vi "SavePixelsVals.vi"(0 "ROI Coordinates out":T1, 5 "Pixel SizeX":dbl, 6 "3D out":T2, 7 "Pixel SizeY":dbl, 8 "Stack length":dbl, 9 "X Start":dbl, 10 "Stack Start":dbl, 11 "error out 2":errorcluster, 12 "X length":dbl, 13 "Y Start":dbl, 14 "Y length":dbl, 15 "Pixel SizeZ":dbl) -> (4 "error out":errorcluster)   [LabVIEW 2011]
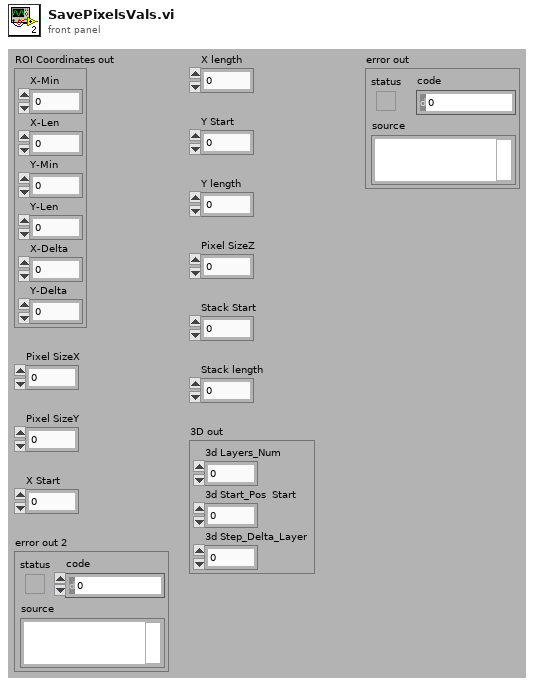
[diagram p1: front panel]
types:
  T1 = cluster{"X-Min":dbl, "X-Len":dbl, "Y-Min":dbl, "Y-Len":dbl, "X-Delta":dbl, "Y-Delta ":dbl}
  T2 = cluster{"3d Layers_Num":dbl, "3d Start_Pos  Start":dbl, "3d Step_Delta_Layer":dbl}
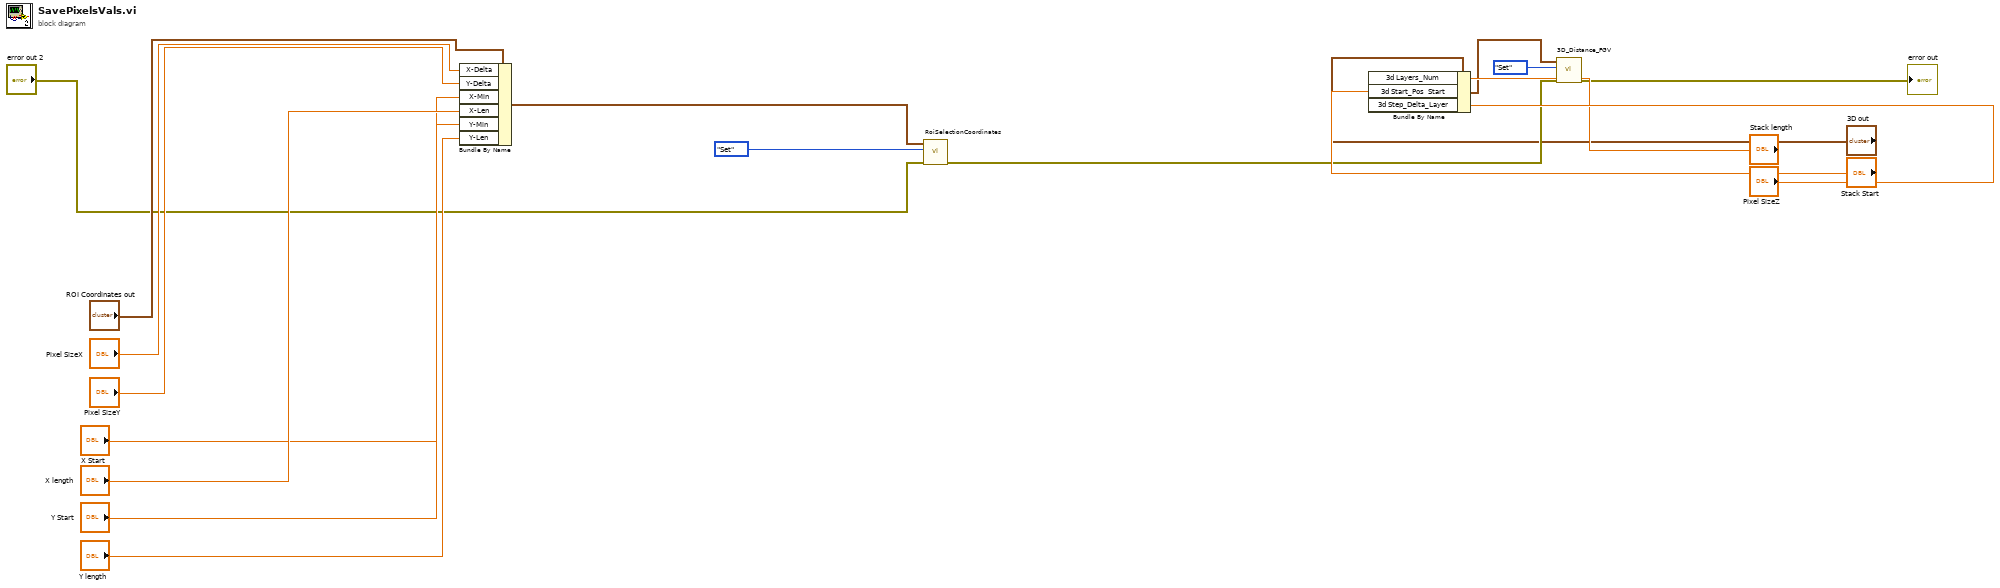
[diagram p0: block diagram]
diagram:
  n1 = Bundle By Name(cluster="ROI Coordinates out", "X-Delta"="Pixel SizeX", "Y-Delta"="Pixel SizeY", "X-Min"="X Start", "X-Len"="X length", "Y-Min"="Y Start", "Y-Len"="Y length") -> (w4:T1)
  n2 = call "RoiSelectionCoordinates.vi"("error in"="error out 2", "FGV_Control"=enum16{"Set", "Get"}."Set", "ROI Coordinates in"=w4) -> ("error out"=w8:errorcluster)  [unwired: 7 in, 1 out]
  n3 = Bundle By Name(cluster="3D out", "3d Layers_Num"="Stack length", "3d Start_Pos  Start"="Stack Start", "3d Step_Delta_Layer"="Pixel SizeZ") -> (w7:T2)
  n4 = call "3D_Distance_FGV.vi"("error in"=w8, "FGV_Control"=enum16{"Set", "Get"}."Set", "3D in"=w7) -> ("error out"=→"error out":errorcluster)  [unwired: 7 in, 1 out]
